vi "Add to Tree.vi"(4 "Child Tag":string, 5 "Child Position":i32, 6 "Display Text Override":string, 7 "Add children? (T)":bool=TRUE, 8 "error in (no error)":errorcluster, 9 "Parent Tag":string, 10 "Tree Manager in":refnum<class "Tree Manager.lvclass">, 11 "Element in":refnum<class "Element.lvclass">) -> (0 "error out":errorcluster, 2 "Tree Manager out":refnum<class "Tree Manager.lvclass">, 3 "Element out":refnum<class "Element.lvclass">)   [LabVIEW 2026, in "VILab.lvlib" / "Element.lvclass"]
uses:
  Element.lvclass
  Tree Manager/Tree Manager.lvclass
  Data Item/Data Item.lvclass
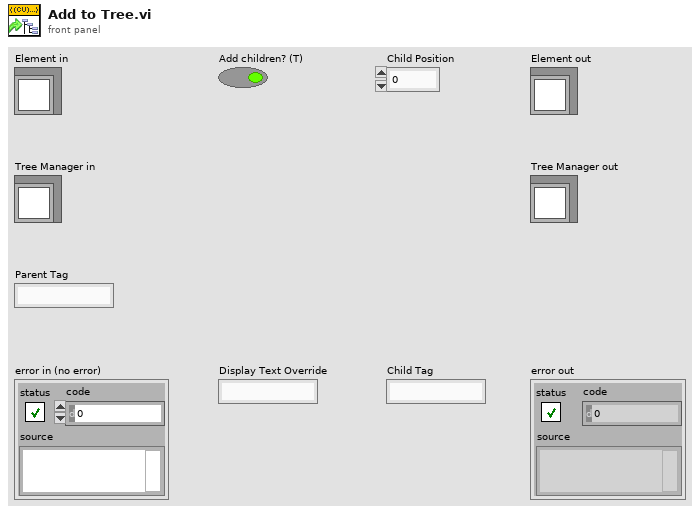
[diagram p1: front panel]
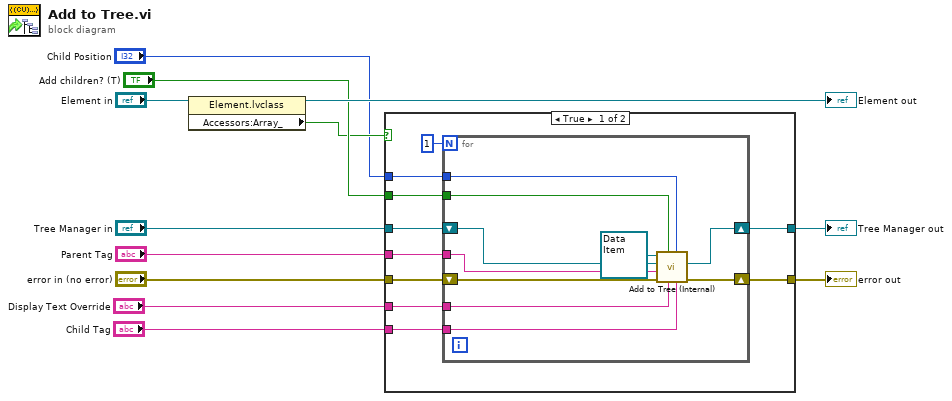
[diagram p0: block diagram]
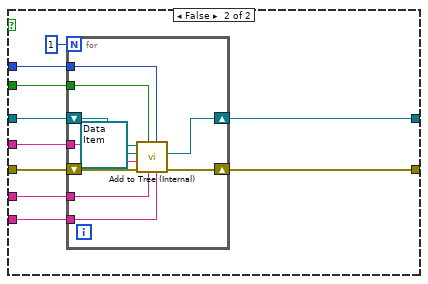
[diagram p2: hidden frame]
diagram:
  n1 = property class="Element.lvclass"(reference="Element in") -> (reference out=→"Element out":refnum<class "Element.lvclass">, "Accessors:Array_"=w4:bool)  [unwired: 1 in, 1 out]
  n2 = case shown="True" w4 {
    tunnel: "error in (no error)" -> [w22 w42]
    tunnel: "Parent Tag" -> [w21 w41]
    tunnel: "Tree Manager in" -> [w20 w40]
    tunnel: [w19 w39] -> w7
    tunnel: [w18 w38] -> w6
    tunnel: "Add children? (T)" -> [w17 w37]
    tunnel: "Child Position" -> [w16 w35]
    tunnel: "Display Text Override" -> [w15 w36]
    tunnel: "Child Tag" -> [w14 w34]
    frame True {
      n3 = for {
        N: 1 -> [_]
        tunnel: w21 -> [w31]
        shift-right: [w28] -> w18
        shift-left: w22 -> [w32]
        shift-right: [w29] -> w19
        shift-left: w20 -> [w30]
        tunnel: w17 -> [w27]
        tunnel: w16 -> [w26]
        tunnel: w15 -> [w25]
        tunnel: w14 -> [w24]
        n4 = call "Add to Tree (Internal).vi"("Child Tag"=w24, "Child Position"=w26, "Display Text Override"=w25, "Add children? (T)"=w27, "error in (no error)"=w32, "Parent Tag"=w31, "Tree Manager in"=w30, "Data Item in"=refnum<class "Data Item.lvclass"> refnum) -> ("error out"=w28:errorcluster, "Tree Manager out"=w29:refnum<class "Tree Manager.lvclass">)  [unwired: 2 out]
      }
    }
    frame False {
      n5 = for {
        N: 1 -> [_]
        tunnel: w41 -> [w51]
        shift-right: [w48] -> w38
        shift-left: w42 -> [w52]
        shift-right: [w49] -> w39
        shift-left: w40 -> [w50]
        tunnel: w37 -> [w47]
        tunnel: w36 -> [w46]
        tunnel: w35 -> [w45]
        tunnel: w34 -> [w44]
        n6 = call "Add to Tree (Internal).vi"("Child Tag"=w44, "Child Position"=w45, "Display Text Override"=w46, "Add children? (T)"=w47, "error in (no error)"=w52, "Parent Tag"=w51, "Tree Manager in"=w50, "Data Item in"=refnum<class "Data Item.lvclass"> refnum) -> ("error out"=w48:errorcluster, "Tree Manager out"=w49:refnum<class "Tree Manager.lvclass">)  [unwired: 2 out]
      }
    }
  }
  "error out" <- w6
  "Tree Manager out" <- w7
